vi "Node - Byte Buffer Read.vi"(8 "error in (no error)":errorcluster, 9 "Buffer Offset In":u64, 10 "Node Local Channels In":T1[](array[typedef]), 11 "Byte Buffer In":refnum<class "Byte Buffer.lvclass">) -> (0 "error out":errorcluster, 1 "Buffer Offset Out":u64, 2 "Node Local Channels Out":T1[](array[typedef]), 3 "Byte Buffer Out":refnum<class "Byte Buffer.lvclass">, 4 "Channel Data Out":dbl[](array[numeric]))   [LabVIEW 2016, in "PXImc Router.lvlib"]
uses:
  PXImc Router.lvlib
  Controls/Node/Node Ch Properties.ctl
  Controls/Data Type.ctl
  <vilib>/NI Veristand/VeriStand Data/Byte Buffer/Byte Buffer.lvclass
  <vilib>/NI Veristand/VeriStand Data/Byte Buffer/Byte Buffer.lvclass/Byte Buffer.ctl
  <vilib>/NI Veristand/VeriStand Data/Byte Buffer/Byte Buffer.Read (Boolean).vi
  <vilib>/NI Veristand/VeriStand Data/Type Conversion/Type Conversion.To Double (Boolean).vi
  <vilib>/NI Veristand/VeriStand Data/Byte Buffer/Byte Buffer.Read (SGL).vi
  <vilib>/NI Veristand/VeriStand Data/Type Conversion/Type Conversion.To Double (SGL).vi
  <vilib>/NI Veristand/VeriStand Data/Byte Buffer/Byte Buffer.Read (DBL).vi
  <vilib>/NI Veristand/VeriStand Data/Byte Buffer/Byte Buffer.Read (I8).vi
  <vilib>/NI Veristand/VeriStand Data/Type Conversion/Type Conversion.To Double (I8).vi
  <vilib>/NI Veristand/VeriStand Data/Byte Buffer/Byte Buffer.Read (I16).vi
  <vilib>/NI Veristand/VeriStand Data/Type Conversion/Type Conversion.To Double (I16).vi
  <vilib>/NI Veristand/VeriStand Data/Byte Buffer/Byte Buffer.Read (I32).vi
  <vilib>/NI Veristand/VeriStand Data/Type Conversion/Type Conversion.To Double (I32).vi
  <vilib>/NI Veristand/VeriStand Data/Byte Buffer/Byte Buffer.Read (I64).vi
  <vilib>/NI Veristand/VeriStand Data/Type Conversion/Type Conversion.To Double (I64).vi
  <vilib>/NI Veristand/VeriStand Data/Byte Buffer/Byte Buffer.Read (U8).vi
  <vilib>/NI Veristand/VeriStand Data/Type Conversion/Type Conversion.To Double (U8).vi
  <vilib>/NI Veristand/VeriStand Data/Byte Buffer/Byte Buffer.Read (U16).vi
  <vilib>/NI Veristand/VeriStand Data/Type Conversion/Type Conversion.To Double (U16).vi
  <vilib>/NI Veristand/VeriStand Data/Byte Buffer/Byte Buffer.Read (U32).vi
  <vilib>/NI Veristand/VeriStand Data/Type Conversion/Type Conversion.To Double (U32).vi
  <vilib>/NI Veristand/VeriStand Data/Byte Buffer/Byte Buffer.Read (U64).vi
  <vilib>/NI Veristand/VeriStand Data/Type Conversion/Type Conversion.To Double (U64).vi
  <vilib>/NI Veristand/VeriStand Data/Byte Buffer/Byte Buffer.Read.Typed String.vi
  <vilib>/NI Veristand/VeriStand Data/Byte Buffer/Byte Buffer.Subset.Get.vi
  <vilib>/NI Veristand/VeriStand Data/Utilities/Utilities.Sizeof.Array.vi
  <vilib>/NI Veristand/VeriStand Data/Utilities/Utilities.Buffer.String.vi
  <vilib>/NI Veristand/VeriStand Data/Byte Buffer/Byte Buffer.Get Buffer Size.vi
  <vilib>/NI Veristand/VeriStand Data/Memory Management/Memory Management.MoveByteBlock.Write (String).vi
  <vilib>/NI Veristand/VeriStand Data/Byte Buffer/Byte Buffer.Get Buffer Pointer.vi
  <vilib>/NI Veristand/VeriStand Data/Utilities/Utilities.Sizeof.Scalar.vi
  <vilib>/NI Veristand/VeriStand Data/Memory Management/Memory Management.Handle Return.vi
  <vilib>/NI Veristand/VeriStand Data/Byte Buffer/Byte Buffer.Get Byte Order.vi
  <vilib>/NI Veristand/VeriStand Data/VeriStand Data.lvlib
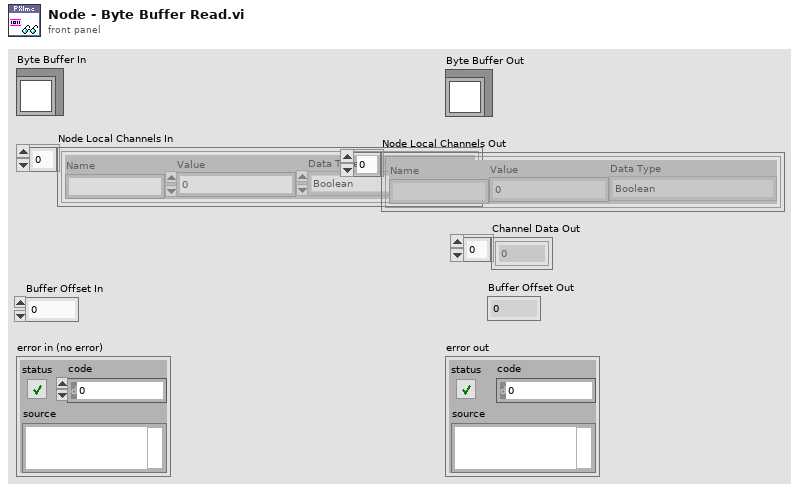
[diagram p1: front panel]
types:
  T1 = typedef "PXImc Router.lvlib/Node Ch Properties.ctl" = cluster{"Name":string, "Value":dbl, "Data Type":T2}
  T2 = typedef "PXImc Router.lvlib/Data Type.ctl" = enum16{"Boolean", "SGL", "DBL", "I8", "I16", "I32", "I64", "U8", "U16", "U32", "U64"}
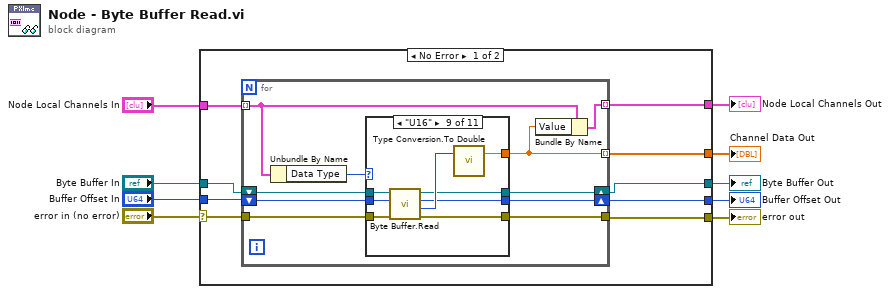
[diagram p0: block diagram]
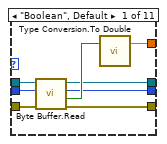
[diagram p2: hidden frame]
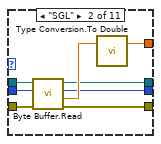
[diagram p3: hidden frame]
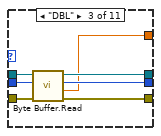
[diagram p4: hidden frame]
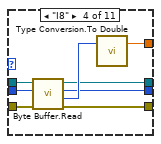
[diagram p5: hidden frame]
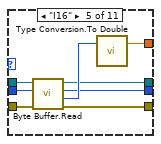
[diagram p6: hidden frame]
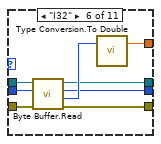
[diagram p7: hidden frame]
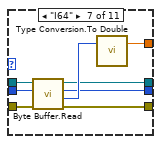
[diagram p8: hidden frame]
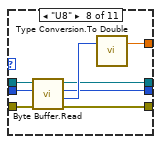
[diagram p9: hidden frame]
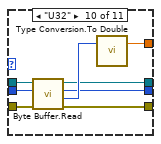
[diagram p10: hidden frame]
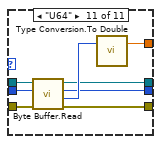
[diagram p11: hidden frame]
diagram:
  n1 = case shown="No Error" "error in (no error)" {
    selector: "error in (no error)" -> [w14 w117]
    tunnel: "Node Local Channels In" -> [w18 w116]
    tunnel: [w17 w117] -> w8
    tunnel: [w16 w118] -> w7
    tunnel: "Byte Buffer In" -> [w15 w118]
    tunnel: [w13 w116] -> w4
    tunnel: [w12 _] -> w3
    tunnel: "Buffer Offset In" -> [w11 _]
    tunnel: [w10 _] -> w1
    frame No Error {
      n2 = for {
        tunnel: [w23] -> w17
        shift-right: [w27] -> w16
        shift-left: w15 -> [w28]
        shift-right: [w24] -> w10
        shift-left: w11 -> [w25]
        tunnel: w14 -> [w26]
        tunnel: w18 -> [w21] mode=indexing
        tunnel: [w20] -> w13 mode=indexing
        tunnel: [w19] -> w12 mode=indexing
        n3 = Unbundle By Name(w21) -> ("Data Type"=w22:T2)
        n4 = case shown="\"U16\"" w22 {
          tunnel: [w35 w43 w45 w58 w66 w74 w82 w90 w98 w106 w114] -> w19
          tunnel: w28 -> [w34 w42 w51 w57 w65 w73 w81 w89 w97 w105 w113]
          tunnel: [w33 w41 w50 w56 w64 w72 w80 w88 w96 w104 w112] -> w27
          tunnel: w26 -> [w32 w40 w49 w55 w63 w71 w79 w87 w95 w103 w111]
          tunnel: w25 -> [w31 w39 w48 w54 w62 w70 w78 w86 w94 w102 w110]
          tunnel: [w30 w38 w47 w53 w61 w69 w77 w85 w93 w101 w109] -> w24
          tunnel: [w29 w37 w46 w52 w60 w68 w76 w84 w92 w100 w108] -> w23
          frame "Boolean", Default {
            n5 = call-poly <vilib>:"Byte Buffer.Read.vi"("error in (no error)"=w32, "buffer offset"=w31, "Byte Buffer in"=w34) -> ("error out"=w29:errorcluster, "value"=w36:bool, "new buffer offset"=w30:u64, "Byte Buffer out"=w33:refnum<class "Byte Buffer.lvclass">)  [unwired: 5 in]
            n6 = call-poly <vilib>:"Type Conversion.To Double.vi"("value in"=w36) -> ("value out"=w35:dbl)  [unwired: 2 in]
          }
          frame "SGL" {
            n7 = call-poly <vilib>:"Byte Buffer.Read.vi"("error in (no error)"=w40, "buffer offset"=w39, "Byte Buffer in"=w42) -> ("error out"=w37:errorcluster, "value"=w44:sgl, "new buffer offset"=w38:u64, "Byte Buffer out"=w41:refnum<class "Byte Buffer.lvclass">)  [unwired: 5 in]
            n8 = call-poly <vilib>:"Type Conversion.To Double.vi"("value in"=w44) -> ("value out"=w43:dbl)  [unwired: 2 in]
          }
          frame "DBL" {
            n9 = call-poly <vilib>:"Byte Buffer.Read.vi"("error in (no error)"=w49, "buffer offset"=w48, "Byte Buffer in"=w51) -> ("error out"=w46:errorcluster, "value"=w45:dbl, "new buffer offset"=w47:u64, "Byte Buffer out"=w50:refnum<class "Byte Buffer.lvclass">)  [unwired: 5 in]
          }
          frame "I8" {
            n10 = call-poly <vilib>:"Byte Buffer.Read.vi"("error in (no error)"=w55, "buffer offset"=w54, "Byte Buffer in"=w57) -> ("error out"=w52:errorcluster, "value"=w59:i8, "new buffer offset"=w53:u64, "Byte Buffer out"=w56:refnum<class "Byte Buffer.lvclass">)  [unwired: 5 in]
            n11 = call-poly <vilib>:"Type Conversion.To Double.vi"("value in"=w59) -> ("value out"=w58:dbl)  [unwired: 2 in]
          }
          frame "I16" {
            n12 = call-poly <vilib>:"Byte Buffer.Read.vi"("error in (no error)"=w63, "buffer offset"=w62, "Byte Buffer in"=w65) -> ("error out"=w60:errorcluster, "value"=w67:i16, "new buffer offset"=w61:u64, "Byte Buffer out"=w64:refnum<class "Byte Buffer.lvclass">)  [unwired: 5 in]
            n13 = call-poly <vilib>:"Type Conversion.To Double.vi"("value in"=w67) -> ("value out"=w66:dbl)  [unwired: 2 in]
          }
          frame "I32" {
            n14 = call-poly <vilib>:"Byte Buffer.Read.vi"("error in (no error)"=w71, "buffer offset"=w70, "Byte Buffer in"=w73) -> ("error out"=w68:errorcluster, "value"=w75:i32, "new buffer offset"=w69:u64, "Byte Buffer out"=w72:refnum<class "Byte Buffer.lvclass">)  [unwired: 5 in]
            n15 = call-poly <vilib>:"Type Conversion.To Double.vi"("value in"=w75) -> ("value out"=w74:dbl)  [unwired: 2 in]
          }
          frame "I64" {
            n16 = call-poly <vilib>:"Byte Buffer.Read.vi"("error in (no error)"=w79, "buffer offset"=w78, "Byte Buffer in"=w81) -> ("error out"=w76:errorcluster, "value"=w83:i64, "new buffer offset"=w77:u64, "Byte Buffer out"=w80:refnum<class "Byte Buffer.lvclass">)  [unwired: 5 in]
            n17 = call-poly <vilib>:"Type Conversion.To Double.vi"("value in"=w83) -> ("value out"=w82:dbl)  [unwired: 2 in]
          }
          frame "U8" {
            n18 = call-poly <vilib>:"Byte Buffer.Read.vi"("error in (no error)"=w87, "buffer offset"=w86, "Byte Buffer in"=w89) -> ("error out"=w84:errorcluster, "value"=w91:u8, "new buffer offset"=w85:u64, "Byte Buffer out"=w88:refnum<class "Byte Buffer.lvclass">)  [unwired: 5 in]
            n19 = call-poly <vilib>:"Type Conversion.To Double.vi"("value in"=w91) -> ("value out"=w90:dbl)  [unwired: 2 in]
          }
          frame "U16" {
            n20 = call-poly <vilib>:"Byte Buffer.Read.vi"("error in (no error)"=w95, "buffer offset"=w94, "Byte Buffer in"=w97) -> ("error out"=w92:errorcluster, "value"=w99:u16, "new buffer offset"=w93:u64, "Byte Buffer out"=w96:refnum<class "Byte Buffer.lvclass">)  [unwired: 5 in]
            n21 = call-poly <vilib>:"Type Conversion.To Double.vi"("value in"=w99) -> ("value out"=w98:dbl)  [unwired: 2 in]
          }
          frame "U32" {
            n22 = call-poly <vilib>:"Byte Buffer.Read.vi"("error in (no error)"=w103, "buffer offset"=w102, "Byte Buffer in"=w105) -> ("error out"=w100:errorcluster, "value"=w107:u32, "new buffer offset"=w101:u64, "Byte Buffer out"=w104:refnum<class "Byte Buffer.lvclass">)  [unwired: 5 in]
            n23 = call-poly <vilib>:"Type Conversion.To Double.vi"("value in"=w107) -> ("value out"=w106:dbl)  [unwired: 2 in]
          }
          frame "U64" {
            n24 = call-poly <vilib>:"Byte Buffer.Read.vi"("error in (no error)"=w111, "buffer offset"=w110, "Byte Buffer in"=w113) -> ("error out"=w108:errorcluster, "value"=w115:u64, "new buffer offset"=w109:u64, "Byte Buffer out"=w112:refnum<class "Byte Buffer.lvclass">)  [unwired: 5 in]
            n25 = call-poly <vilib>:"Type Conversion.To Double.vi"("value in"=w115) -> ("value out"=w114:dbl)  [unwired: 2 in]
          }
        }
        n26 = Bundle By Name(cluster=w21, "Value"=w19) -> (w20:T1)
      }
    }
    frame Error {
    }
  }
  "error out" <- w8
  "Byte Buffer Out" <- w7
  "Node Local Channels Out" <- w4
  "Channel Data Out" <- w3
  "Buffer Offset Out" <- w1
